vi "DataPlayback.vi"(8 "error in (no error)":errorcluster, 9 "Datalength":i32=3600, 10 "Controller Name":string="F4", 11 "file path":path) -> (0 "error out":errorcluster, 3 "Array":waveform(dbl)[](array[waveform]))   [LabVIEW 2010]
doc: "Use this template to build a VI to use as a subVI."
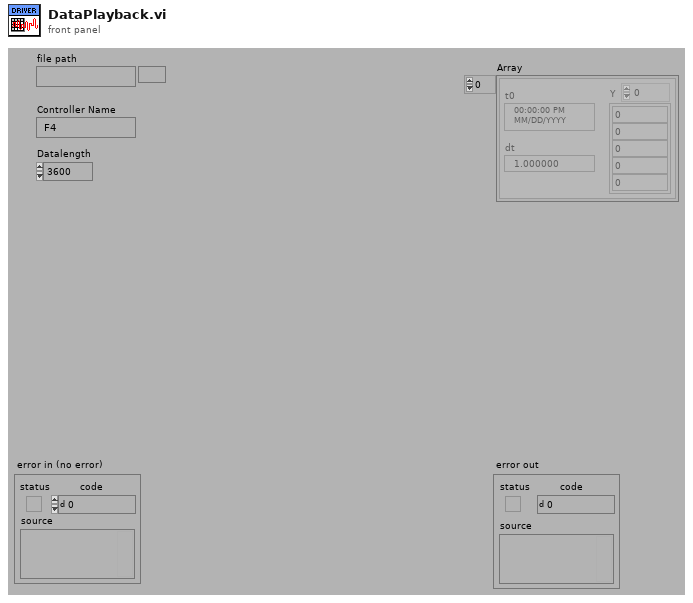
[diagram p1: front panel]
types:
  T1 = enum16{"open", "open or create", "create or replace", "create", "open (read-only)"}
  T2 = typedef "Path InitPaths__FS.ctl" = cluster{"Ctrller CFG":path, "INI":path, "Profile":path, "EventLog":path, "Data":path}
  T3 = typedef "Controller Configuration__CHC.ctl" = cluster{"Ctrller Type":T4, "Ctrller Name":string, "Ctrller Addr":string, "Server IP":string, "Conn Result":string, "Port":string, "Baud":dbl}
  T4 = typedef "Controller Configuration__Ctrller Type.ctl" = enum16{"F4S/D", "Synergy"}
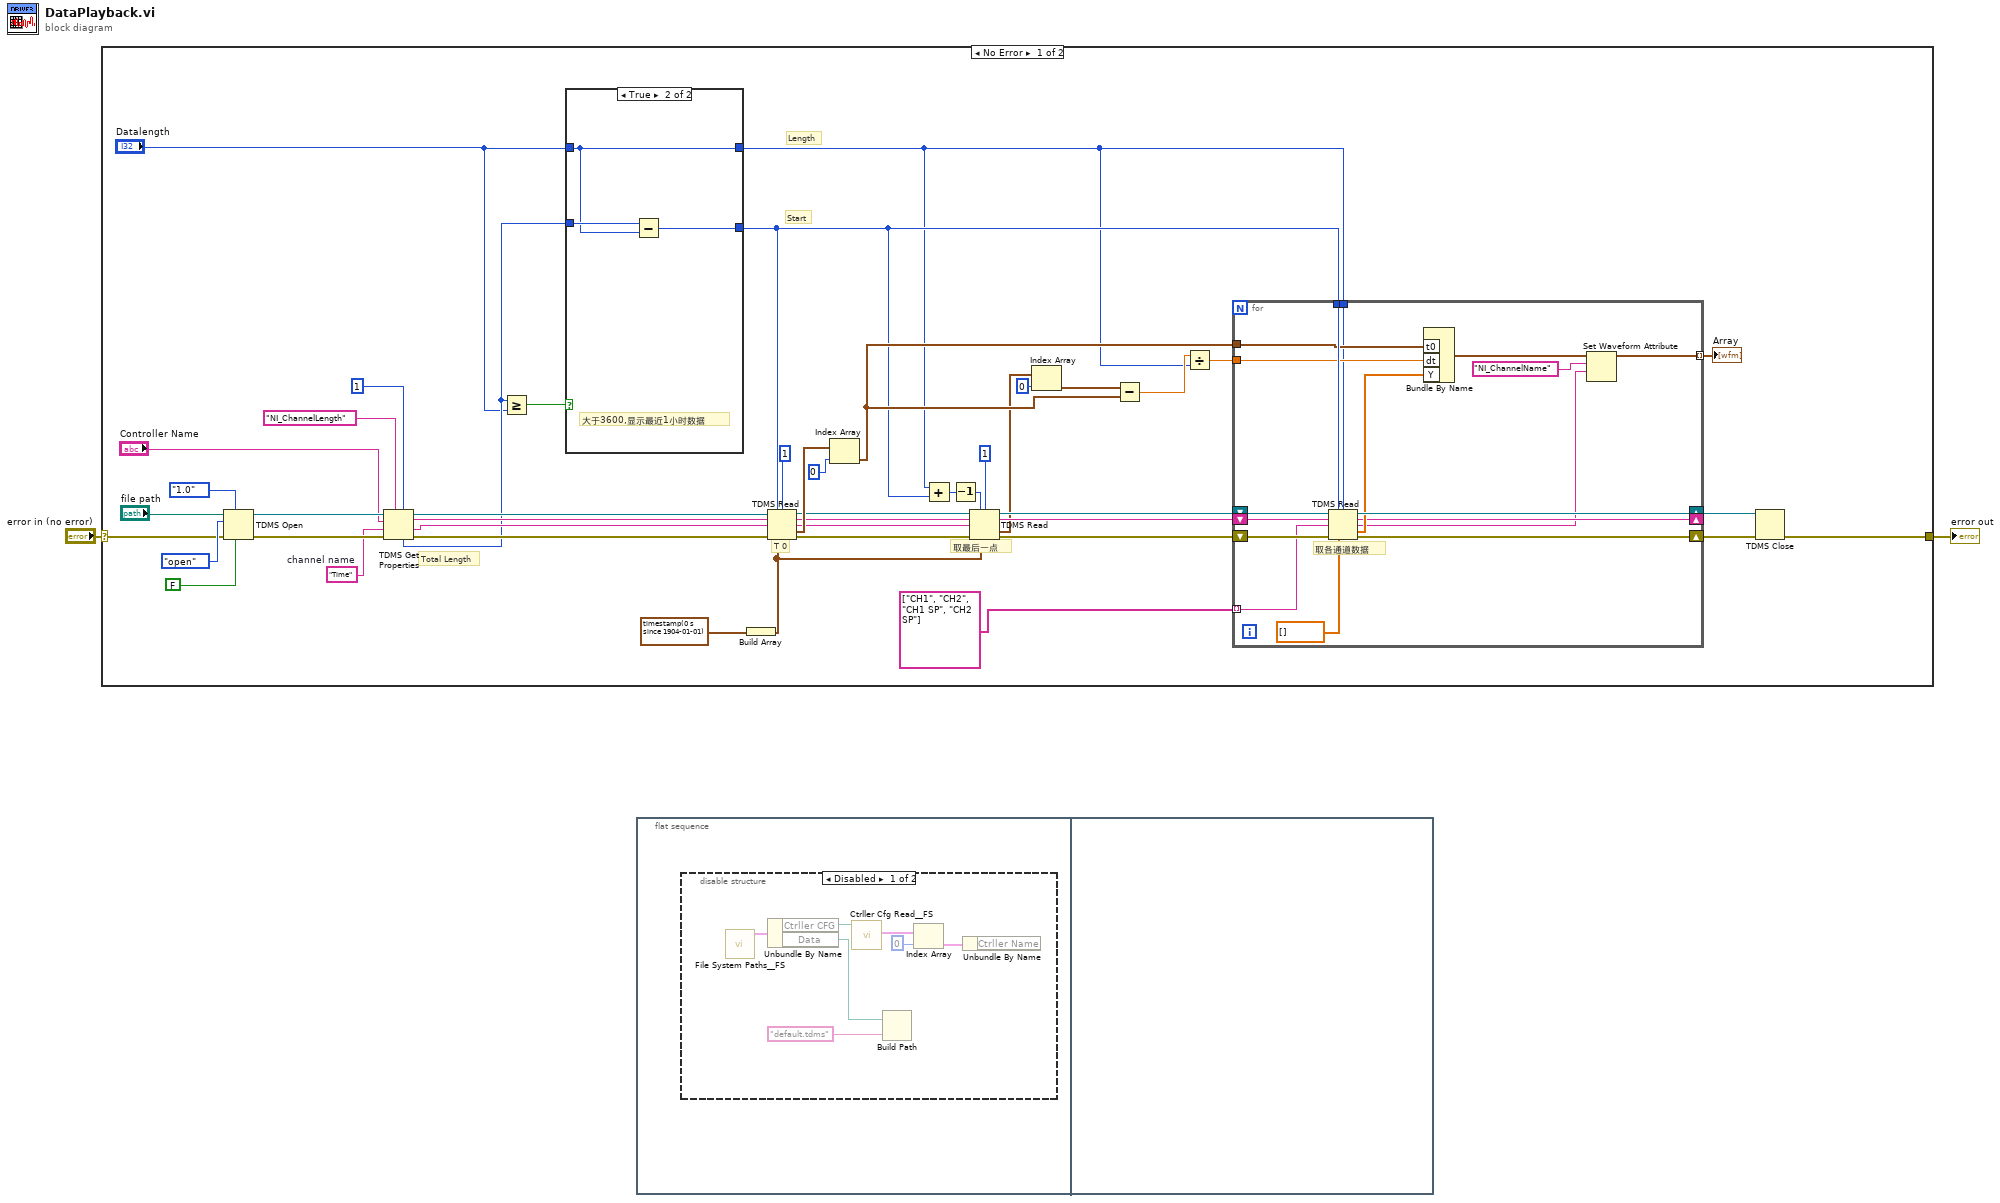
[diagram p0: block diagram]
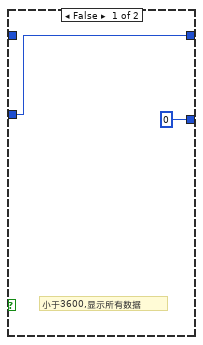
[diagram p3: hidden frame]
diagram:
  n1 = case shown="No Error" "error in (no error)" {
    selector: "error in (no error)" -> [w13 w71]
    tunnel: [w15 w71] -> w1
    frame No Error {
      w24 = "Time"  # channel name
      # "Length"
      # "Start"
      # "Total Length"
      # "取最后一点"
      # "T 0"
      n2 = TDMS Open(6:FALSE ("disable buffering? (T)"), 7:enum16{"1.0", "2.0"}."1.0" ("file format version (2.0)"), 8:w13, 10:T1."open" ("operation (0:open)"), 11:"file path") -> (0:w38:errorcluster, 3:w40:refnum<k34>)  [unwired: 1 in]
      n3 = TDMS Get Properties(5:1 ("index"), 7:"NI_ChannelLength" ("property name"), 8:w38, 9:w24, 10:"Controller Name", 11:w40) -> (0:w37:errorcluster, 1:w25:string, 2:w33:string, 3:w39:refnum<k34>, 4:w11:i32)  [unwired: 1 out]
      n4 = Greater Or Equal?(x=w11, y="Datalength") -> (x >= y?=w12:bool)
      n5 = case shown="True" w12 {
        tunnel: [0 w51] -> w9
        tunnel: [w49 w52] -> w5
        tunnel: w11 -> [w49 w53]
        tunnel: "Datalength" -> [_ w52]
        frame False {
          # "小于3600,显示所有数据"
        }
        frame True {
          # "大于3600,显示最近1小时数据"
          n6 = Subtract(x=w53, y=w52) -> (x-y=w51:i32)
        }
      }
      n7 = Build Array(timestamp(0 s since 1904-01-01) ("current time")) -> (w23:timestamp[])
      n8 = TDMS Read(0:w39, 1:w9, 2:i64 1 ("count (-1: all)"), 5:w33, 7:w25, 11:w37, 12:w23) -> (4:w32:refnum<k34>, 6:w29:string, 8:w31:string, 10:w43:timestamp[], 15:w30:errorcluster)  [unwired: 1 out]
      n9 = Index Array(array=w43, index=0) -> (element=w42:timestamp)
      n10 = Add(x=w5, y=w9) -> (x+y=w8:i32)
      n11 = Decrement(x=w8) -> (x-1=w7:i32)
      n12 = TDMS Read(0:w32, 1:w7, 2:i64 1 ("count (-1: all)"), 5:w29, 7:w31, 11:w30, 12:w23) -> (4:w27:refnum<k34>, 6:w28:string, 10:w20:timestamp[], 15:w26:errorcluster)  [unwired: 2 out]
      n13 = Index Array(array=w20, index=0) -> (element=w18:timestamp)
      n14 = Subtract(x=w18, y=w42) -> (x-y=w41:dbl)
      n15 = Divide(x=w41, y=w5) -> (x/y=w6:dbl)
      n16 = for {
        tunnel: w9 -> [w67]
        tunnel: w42 -> [w64]
        tunnel: w6 -> [w63]
        tunnel: [w62] -> w4 mode=indexing
        tunnel: w5 -> [w59]
        shift-right: [w70] -> w16
        shift-left: w27 -> [w57]
        shift-right: [w60] -> _
        shift-left: w28 -> [w58]
        shift-right: [w69] -> w17
        shift-left: w26 -> [w56]
        tunnel: string[] ["CH1", "CH2", "CH1 SP", "CH2 SP"] ("channel name(s) in (Untitled)") -> [w54] mode=indexing
        # "取各通道数据"
        n17 = TDMS Read(0:w57, 1:w67, 2:w59, 5:w58, 7:w54, 11:w56, 12:dbl[] [] ("appended array")) -> (4:w70:refnum<k34>, 6:w60:string, 8:w55:string, 10:w66:dbl[], 15:w69:errorcluster)  [unwired: 1 out]
        n18 = Bundle By Name("t0"=w64, "dt"=w63, "Y"=w66) -> (w65:waveform(dbl))  [unwired: 1 in]
        n19 = Set Waveform Attribute(5:w55, 6:"NI_ChannelName" ("name"), 7:w65) -> (3:w62:waveform(dbl))  [unwired: 1 in, 2 out]
      }
      "Array" <- w4
      n20 = TDMS Close(8:w17, 11:w16) -> (0:w15:errorcluster)  [unwired: 1 out]
    }
    frame Error {
    }
  }
  "error out" <- w1
  n21 = flat-sequence {
    frame #0 {
      n22 = disable-structure shown="Disabled" {
        frame Disabled {
          n23 = call "File System Paths__FS.vi"() -> ("FilePaths"=w77:T2)  [unwired: 9 in, 2 out]
          n24 = Unbundle By Name(w77) -> ("Ctrller CFG"=w78:path, "Data"=w72:path)
          n25 = call "Ctrller Cfg Read__FS.vi"("Path In"=w78) -> ("Ctrllers"=w76:T3[])  [unwired: 8 in, 2 out]
          n26 = Build Path(base path=w72, name or relative path="default.tdms") -> ()  [unwired: 1 out]
          n27 = Index Array(array=w76, index=0) -> (element=w74:T3)
          n28 = Unbundle By Name(w74) -> ()  [unwired: 1 out]
        }
        frame Enabled {
        }
      }
    }
    frame #1 {
    }
  }
